vi "Tosca-Save Multrig Settings.vi"(0 "Table":cluster{string, string, string, string}[](array[cluster]), 7 "Apply defaults":bool) -> ()   [LabVIEW 2020]
uses:
  epl-vi-lib/Utility VIs/File IO VIs/Configuration File Wrapper VIs/Config-Read Key (string).vi
  epl-vi-lib/Utility VIs/File IO VIs/Configuration File Wrapper VIs/Config-Write Key (string).vi
  TTL VIs/Device Classes/Base Class/TTLControlledDevice.lvclass
  epl-vi-lib/Utility VIs/Type Defs/TCP Params.ctl
  D:/Development/epl-vi-lib/Koop/KObject Class/KObject.lvclass
  D:/Development/epl-tosca/LV Source/TTL VIs/Device Classes/Base Class/TTLControlledDevice.lvclass
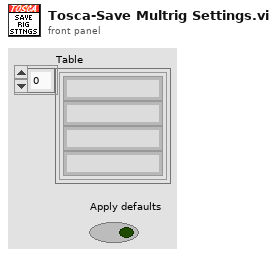
[diagram p1: front panel]
types:
  T1 = typedef "TCP Params.ctl" = cluster{"IP Address":string, "Port":i32}
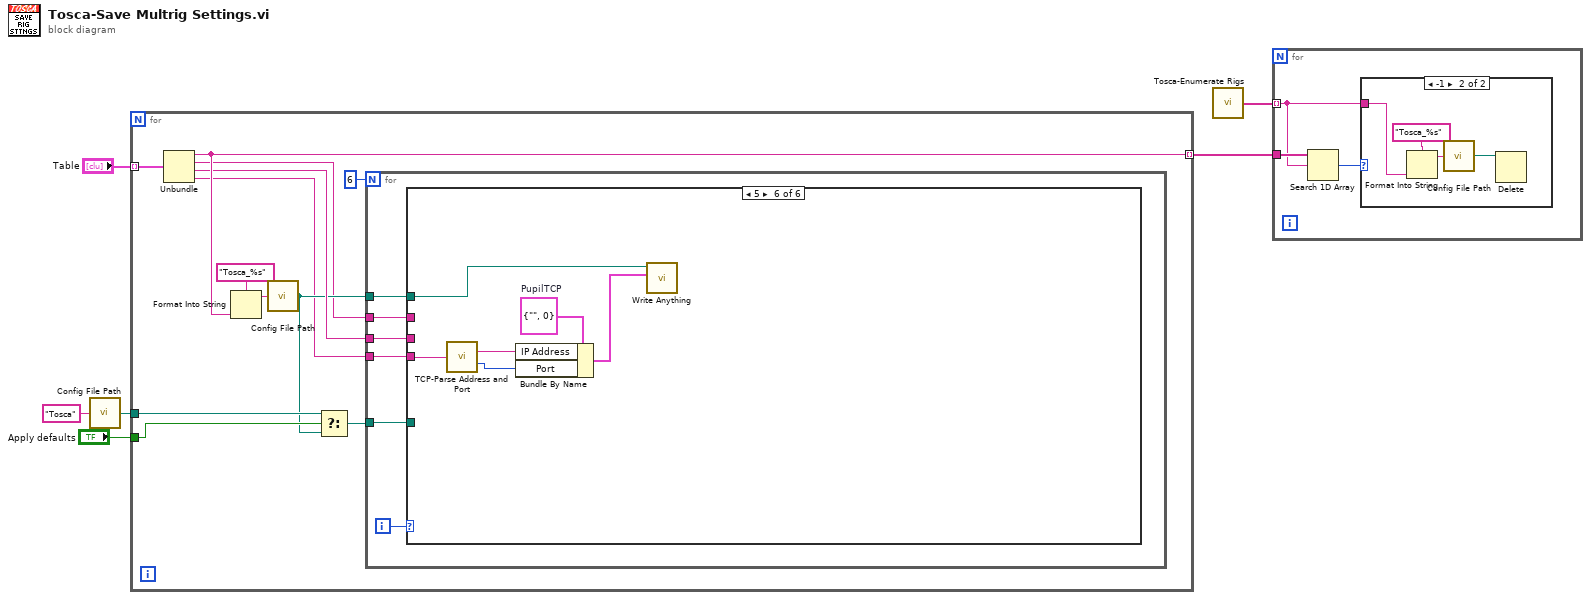
[diagram p0: block diagram]
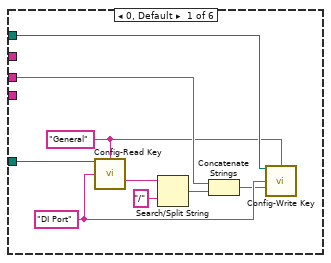
[diagram p2: hidden frame]
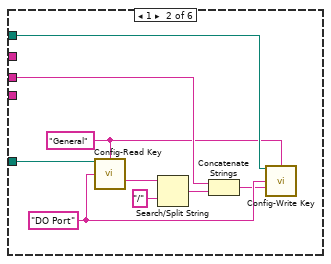
[diagram p3: hidden frame]
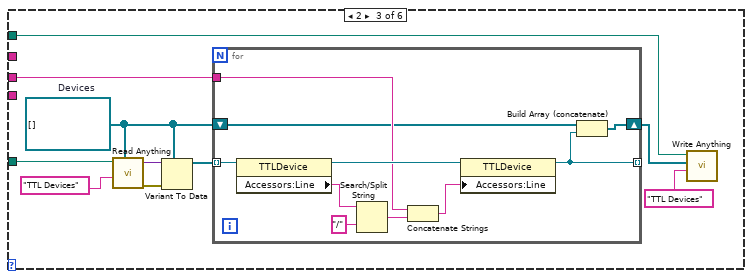
[diagram p4: hidden frame]
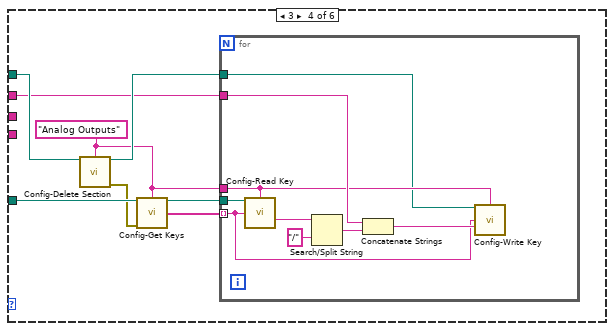
[diagram p5: hidden frame]
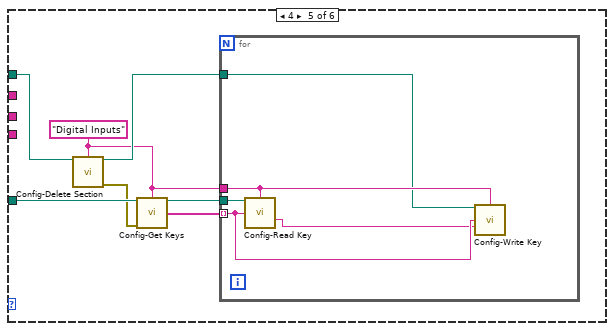
[diagram p6: hidden frame]
diagram:
  n1 = call "Config File Path.vi"("AppName"="Tosca") -> ("Default config file name"=w1:path)
  n2 = for {
    tunnel: "Table" -> [w16] mode=indexing
    tunnel: "Apply defaults" -> [w13]
    tunnel: [w15] -> w3 mode=indexing
    tunnel: w1 -> [w14]
    n3 = Unbundle(w16) -> (w15:string, w9:string, w11:string, w7:string)
    n4 = Format Into String(format string="Tosca_%s", w15) -> (resulting string=w17:string)  [unwired: 2 in, 1 out]
    n5 = call "Config File Path.vi"("AppName"=w17) -> ("Default config file name"=w10:path)
    n6 = Select(t=w14, s=w13, f=w10) -> (s? t:f=w12:path)
    n7 = for {
      N: 6 -> [_]
      tunnel: w12 -> [w24]
      tunnel: w11 -> [w23]
      tunnel: w10 -> [w22]
      tunnel: w9 -> [w21]
      tunnel: w7 -> [w19]
      i -> [w20]
      n8 = case shown="5" w20 {
        tunnel: w24 -> [w33 w42 w51 w70 w86 _]
        tunnel: w23 -> [w29 w38 w47 _ _ _]
        tunnel: w22 -> [w28 w37 w45 w67 w83 w93]
        tunnel: w21 -> [_ _ _ w65 _ _]
        tunnel: w19 -> [_ _ _ _ _ w97]
        frame 0, Default {
          w27 = "DI Port" ("key")
          w25 = "General" ("section")
          n9 = call-poly "Config-Read Key.vi"("configuration file path"=w33, "section"=w25, "key"=w27) -> ("value"=w30:string)  [unwired: 9 in, 3 out]
          n10 = Search/Split String(string=w30, search string/char (-)="/") -> (match + rest of string=w32:string)  [unwired: 1 in, 2 out]
          n11 = Concatenate Strings(w29, w32) -> (w26:string)
          n12 = call-poly "Config-Write Key.vi"("configuration file path"=w28, "section"=w25, "key"=w27, "value"=w26) -> ()  [unwired: 9 in, 3 out]
        }
        frame 1 {
          w36 = "DO Port" ("key")
          w34 = "General" ("section")
          n13 = call-poly "Config-Read Key.vi"("configuration file path"=w42, "section"=w34, "key"=w36) -> ("value"=w39:string)  [unwired: 9 in, 3 out]
          n14 = Search/Split String(string=w39, search string/char (-)="/") -> (match + rest of string=w41:string)  [unwired: 1 in, 2 out]
          n15 = Concatenate Strings(w38, w41) -> (w35:string)
          n16 = call-poly "Config-Write Key.vi"("configuration file path"=w37, "section"=w34, "key"=w36, "value"=w35) -> ()  [unwired: 9 in, 3 out]
        }
        frame 2 {
          w44 = refnum<class "TTLControlledDevice.lvclass">[] []  # Devices
          n17 = call "Read Anything.vi"("Type of Anything"=w44, "Section Name (Name of \"Type of Anything\")"="TTL Devices" ("Section Name (Name of \"Type of Anything\")"), "Path (dialog)"=w51) -> ("Error Out"=w50:errorcluster, "Anything"=w49:variant)  [unwired: 6 in, 1 out]
          n18 = Variant To Data(error in=w50, type=w44, Variant=w49) -> (data=w48:refnum<class "TTLControlledDevice.lvclass">[])  [unwired: 1 out]
          n19 = for {
            tunnel: w48 -> [w62] mode=indexing
            tunnel: w47 -> [w57]
            tunnel: [w54] -> _ mode=indexing
            shift-right: [w53] -> w43
            shift-left: w44 -> [w55]
            n20 = property class="TTLDevice"(reference=w62) -> (reference out=w61:refnum<class "TTLControlledDevice.lvclass">, "Accessors:Line"=w58:string)  [unwired: 1 in, 1 out]
            n21 = Search/Split String(string=w58, search string/char (-)="/") -> (match + rest of string=w60:string)  [unwired: 1 in, 2 out]
            n22 = Concatenate Strings(w57, w60) -> (w56:string)
            n23 = property class="TTLDevice"(reference=w61, "Accessors:Line"=w56) -> (reference out=w54:refnum<class "TTLControlledDevice.lvclass">)  [unwired: 1 in, 1 out]
            n24 = Build Array (concatenate)(w55, w54) -> (w53:refnum<class "TTLControlledDevice.lvclass">[])
          }
          n25 = call "Write Anything.vi"("Section Name (Name of \"Anything\")"="TTL Devices" ("Section Name (Name of \"Type of Anything\")"), "Anything"=w43, "Path (dialog)"=w45) -> ()  [unwired: 7 in, 2 out]
        }
        frame 3 {
          w63 = "Analog Outputs" ("section")
          n26 = call "Config-Delete Section.vi"("configuration file path"=w67, "section"=w63) -> ("file path"=w66:path, "error out"=w64:errorcluster)  [unwired: 12 in]
          n27 = call "Config-Get Keys.vi"("configuration file path"=w70, "section"=w63, "error in (no error)"=w64) -> ("file path"=w68:path, "key names"=w69:string[])  [unwired: 10 in, 1 out]
          n28 = for {
            tunnel: w69 -> [w73] mode=indexing
            tunnel: w66 -> [w71]
            tunnel: w63 -> [w72]
            tunnel: w68 -> [w77]
            tunnel: w65 -> [w75]
            n29 = call-poly "Config-Read Key.vi"("configuration file path"=w77, "section"=w72, "key"=w73) -> ("value"=w76:string)  [unwired: 9 in, 3 out]
            n30 = Search/Split String(string=w76, search string/char (-)="/") -> (match + rest of string=w79:string)  [unwired: 1 in, 2 out]
            n31 = Concatenate Strings(w75, w79) -> (w74:string)
            n32 = call-poly "Config-Write Key.vi"("configuration file path"=w71, "section"=w72, "key"=w73, "value"=w74) -> ()  [unwired: 9 in, 3 out]
          }
        }
        frame 4 {
          w80 = "Digital Inputs" ("section")
          n33 = call "Config-Delete Section.vi"("configuration file path"=w83, "section"=w80) -> ("file path"=w82:path, "error out"=w81:errorcluster)  [unwired: 12 in]
          n34 = call "Config-Get Keys.vi"("configuration file path"=w86, "section"=w80, "error in (no error)"=w81) -> ("file path"=w84:path, "key names"=w85:string[])  [unwired: 10 in, 1 out]
          n35 = for {
            tunnel: w85 -> [w90] mode=indexing
            tunnel: w82 -> [w88]
            tunnel: w80 -> [w89]
            tunnel: w84 -> [w91]
            n36 = call-poly "Config-Read Key.vi"("configuration file path"=w91, "section"=w89, "key"=w90) -> ("value"=w87:string)  [unwired: 9 in, 3 out]
            n37 = call-poly "Config-Write Key.vi"("configuration file path"=w88, "section"=w89, "key"=w90, "value"=w87) -> ()  [unwired: 9 in, 3 out]
          }
        }
        frame 5 {
          w96 = T1 {"IP Address"="", "Port"=0}  # PupilTCP
          n38 = call "TCP-Parse Address and Port.vi"("Address in"=w97) -> ("Address"=w95:string, "Port"=w94:i32)  [unwired: 12 in, 1 out]
          n39 = Bundle By Name(cluster=w96, "IP Address"=w95, "Port"=w94) -> (w92:T1)
          n40 = call "Write Anything.vi"("Anything"=w92, "Path (dialog)"=w93) -> ()  [unwired: 8 in, 2 out]
        }
      }
    }
  }
  n41 = call "Tosca-Enumerate Rigs.vi"() -> ("Rigs"=w2:string[])  [unwired: 15 in]
  n42 = for {
    tunnel: w2 -> [w98] mode=indexing
    tunnel: w3 -> [w100]
    n43 = Search 1D Array(1D array=w100, element=w98) -> (index of element=w99:i32)  [unwired: 1 in]
    n44 = case shown="-1" w99 {
      tunnel: w98 -> [_ w103]
      frame 0, Default {
      }
      frame -1 {
        n45 = Format Into String(format string="Tosca_%s", w103) -> (resulting string=w104:string)  [unwired: 2 in, 1 out]
        n46 = call "Config File Path.vi"("AppName"=w104) -> ("Default config file name"=w102:path)
        n47 = Delete(path (use dialog)=w102) -> ()  [unwired: 4 in, 3 out]
      }
    }
  }
